vi "Revision Query.vi"(8 "error in (no error)":errorcluster, 11 "VISA resource name":refnum<visa-resource-name>) -> (0 "error out":errorcluster, 1 "Instr Serial Number":string, 2 "Instr Firmware Revision":string, 3 "VISA resource name out":refnum<visa-resource-name>, 4 "Instr Model Number":string, 5 "Instrument Driver Revision":string)   [LabVIEW 2019, in "Lake Shore 325.lvlib"]
doc: "Queries the current instrument firmware revision and instrument driver revision.\n\nFor detailed driver information including modification history, refer to the Readme file."
uses:
  Lake Shore 325.lvlib
  Instance           2 22Saved   Revision Query .vi
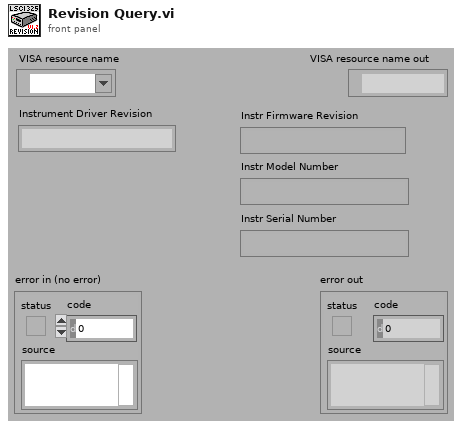
[diagram p1: front panel]
types:
  T1 = enum32{"invalid app kind", "Development System", "Run Time System", "Student Edition", "Embedded LabVIEW", "Evaluation", "Custom"}
  T2 = cluster{"Major":u16, "Minor":u16, "Fix":u16, "Build":u16}
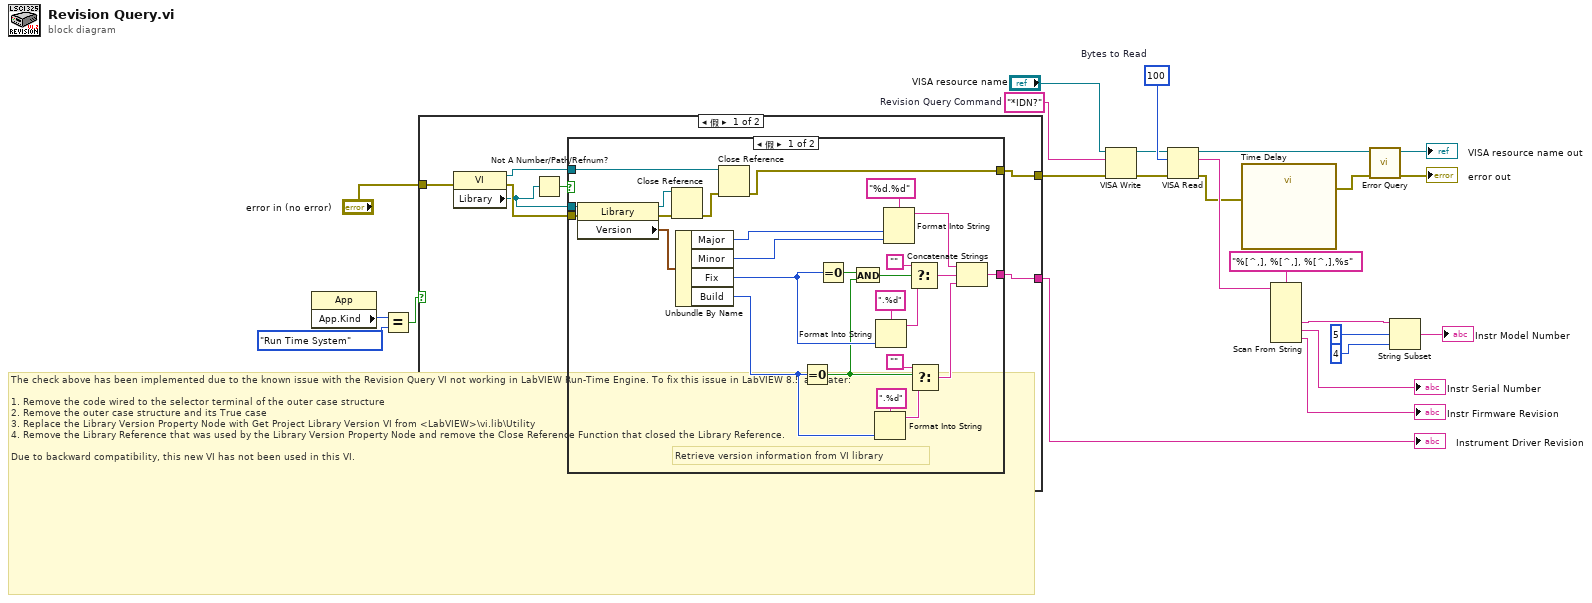
[diagram p0: block diagram]
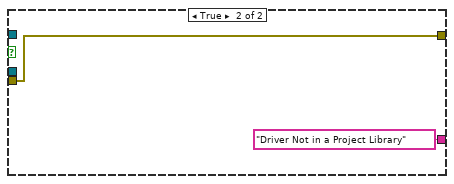
[diagram p2: hidden frame]
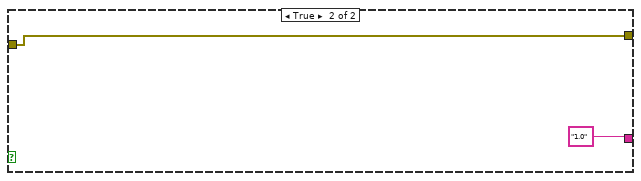
[diagram p3: hidden frame]
diagram:
  w20 = "*IDN?"  # Revision Query Command
  w23 = u32 100  # Bytes to Read
  # "The check above has been implemented due to the known issue with the Revision Query VI not working in LabVIEW Run-Time Engine. To fix this issue in LabVIEW 8.5 and later:\n\n1. Remove the code wired to the selector terminal of the outer case structure\n2. Remove the outer case structure and its True case\n3. Replace the Library Version Property Node with Get Project Library Version VI from <LabVIEW>\\vi.lib\\Utility\n4. Remove the Library Reference that was used by the Library Version Property Node and remove the Close Reference Function that closed the Library Reference.\n\nDue to backward compatibility, this new VI has not been used in this VI."
  n1 = property class="App"() -> ("App.Kind"=w6:T1)  [unwired: 2 in, 2 out]
  n2 = Equal?(x=w6, y=T1."Run Time System") -> (x = y?=w7:bool)
  n3 = case shown="假" w7 {
    tunnel: "error in (no error)" -> [w31 w61]
    tunnel: [w26 "1.0"] -> w9
    tunnel: [w25 w61] -> w8
    frame False {
      n4 = property on="Property Node" class="VI"(error in=w31) -> (reference out=w27:refnum<vi>, error out=w30:errorcluster, "Library"=w29:refnum<vi>)  [unwired: 1 in]
      n5 = Not A Number/Path/Refnum?(number/path/refnum=w29) -> (NaN/Path/Refnum?=w28:bool)
      n6 = case shown="假" w28 {
        tunnel: [w36 w58] -> w25
        tunnel: [w35 "Driver Not in a Project Library"] -> w26
        tunnel: w30 -> [w34 w58]
        tunnel: w29 -> [w33 _]
        tunnel: w27 -> [w32 _]
        frame False {
          # "Retrieve version information from VI library"
          n7 = property on="Property Node" class="Library"(reference=w33, error in=w34) -> (reference out=w56:refnum<vi>, error out=w57:errorcluster, "Version"=w54:T2)
          n8 = Close Reference(reference=w56, error in (no error)=w57) -> (error out=w55:errorcluster)
          n9 = Unbundle By Name(w54) -> ("Major"=w43:u16, "Minor"=w42:u16, "Fix"=w40:u16, "Build"=w41:u16)
          n10 = Close Reference(reference=w32, error in (no error)=w55) -> (error out=w36:errorcluster)
          n11 = Equal To 0?(x=w41) -> (x = 0?=w38:bool)
          n12 = Equal To 0?(x=w40) -> (x = 0?=w39:bool)
          n13 = And(x=w39, y=w38) -> (x .and. y?=w37:bool)
          n14 = Format Into String(format string=".%d", w41) -> (resulting string=w47:string)  [unwired: 2 in, 1 out]
          n15 = Format Into String(format string=".%d", w40) -> (resulting string=w51:string)  [unwired: 2 in, 1 out]
          n16 = Format Into String(format string="%d.%d", w43, w42) -> (resulting string=w49:string)  [unwired: 2 in, 1 out]
          n17 = Select(t="" ("Empty String Constant"), s=w37, f=w51) -> (s? t:f=w48:string)
          n18 = Select(t="" ("Empty String Constant"), s=w38, f=w47) -> (s? t:f=w44:string)
          n19 = Concatenate Strings(w49, w48, w44) -> (w35:string)
        }
        frame True {
        }
      }
    }
    frame True {
    }
  }
  "Instrument Driver Revision" <- w9
  n20 = VISA Write(VISA resource name="VISA resource name", write buffer=w20, error in (no error)=w8) -> (VISA resource name out=w22:refnum<visa-resource-name>, error out=w21:errorcluster)  [unwired: 1 out]
  n21 = VISA Read(VISA resource name=w22, byte count=w23, error in (no error)=w21) -> (VISA resource name out=w19:refnum<visa-resource-name>, read buffer=w15:string, error out=w12:errorcluster)  [unwired: 1 out]
  n22 = call "Time Delay"("error in (no error)"=w12) -> ("error out"=w11:errorcluster)  [unwired: 10 in]
  n23 = Scan From String(format string="%[^,], %[^,], %[^,],%s", input string=w15) -> (output 2=w1:string, output 3=→"Instr Serial Number":string, output 4=→"Instr Firmware Revision":string)  [unwired: 7 in, 3 out]
  n24 = call "Error Query.vi"("error in (no error)"=w11, "VISA resource name"=w19) -> ("error out"=→"error out":errorcluster, "VISA resource name out"=→"VISA resource name out":refnum<visa-resource-name>)  [unwired: 7 in, 1 out]
  n25 = String Subset(string=w1, offset (0)=5, length (rest)=4) -> (substring=→"Instr Model Number":string)
